vi "run.vi"(8 "error in (no error)":errorcluster, 11 "ScanModeDL091001Scaffold in":refnum<class "ImagingModeDL091001Scaffold.lvclass">) -> (0 "error out":errorcluster, 3 "ScanModeDL091001Scaffold out":refnum<class "ImagingModeDL091001Scaffold.lvclass">)   [LabVIEW 2010, in "ImagingModeDL091001Scaffold.lvclass"]
uses:
  ImagingModeDL091001Scaffold.lvclass
  internal_triggers_enum.ctl
  GenericImagingMode/GenericImagingMode/trigger_enum.ctl
  GenericImagingMode/GenericImagingMode/GenericImagingMode.lvclass
  Trajectory/GenericTrajectory/GenericTrajectory/GenericTrajectory.lvclass
  common/classes/ErrorController/ErrorController/class_data.vi
  common/classes/ErrorController/ErrorController/ErrorController.lvclass
panel:
  out "last trigger":T1
  out "statechart\nerror 2":errorcluster
  out "stage machine counter":i32
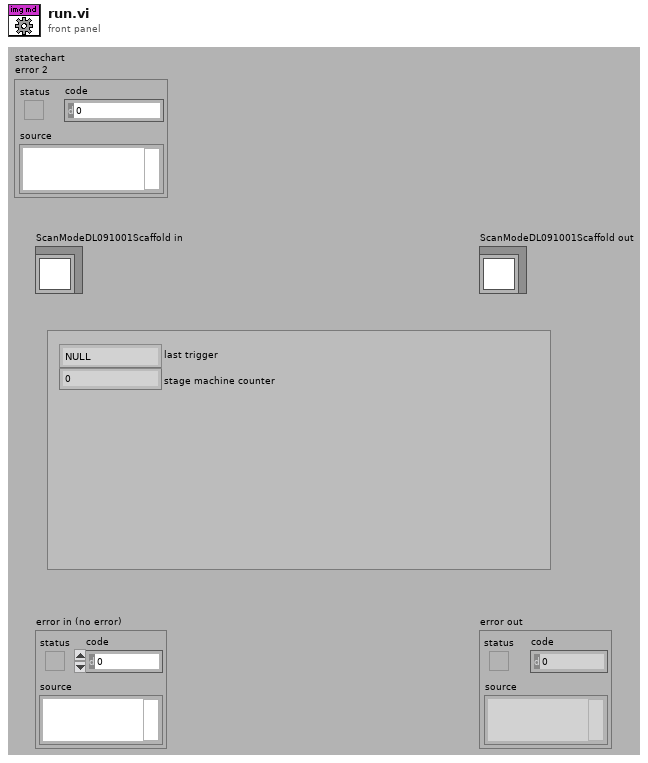
[diagram p1: front panel]
types:
  T1 = typedef "ImagingModeDL091001Scaffold.lvclass/internal_triggers_enum.ctl" = enum16{"NULL", "initialise", "terminate", "start sweep", "stop sweep", "update", "proceed", "draw overlay", "attach observer", "detach observer", "finish sweep"}
  T2 = typedef "GenericImagingMode.lvclass/trigger_enum.ctl" = enum16{"NULL", "proceed"}
  T3 = typedef "top-level_component_type_enum.ctl" = enum16{"undefined", "ImagingMode", "ScanHead", "DAQ", "ImageAssembler", "Display", "DataCollection", "Analyser", "Stimulator", "ExperimentController", "Instrument", "Stage"}
  T4 = typedef "main_trigger_enum.ctl" = enum16{"NULL", "initialise", "terminate", "start", "stop", "change objective", "change experimentController", "change imagingMode", "save notebook", "started saving", "finished saving", "expCtr ready", "expCtr missing", "imgMd ready", "imgMd missing", "scanHd ready", "scanHd missing", "DAQ ready", "DAQ missing", "imgAsm ready", "imgAsm missing", "dataColl ready", "dataColl missing", "display ready", "display missing", "analysr ready", "analysr missing", "instrmnt ready", "instrmnt missing", "stimltr ready", "stimltr missing", "stage ready", "stage missing"}
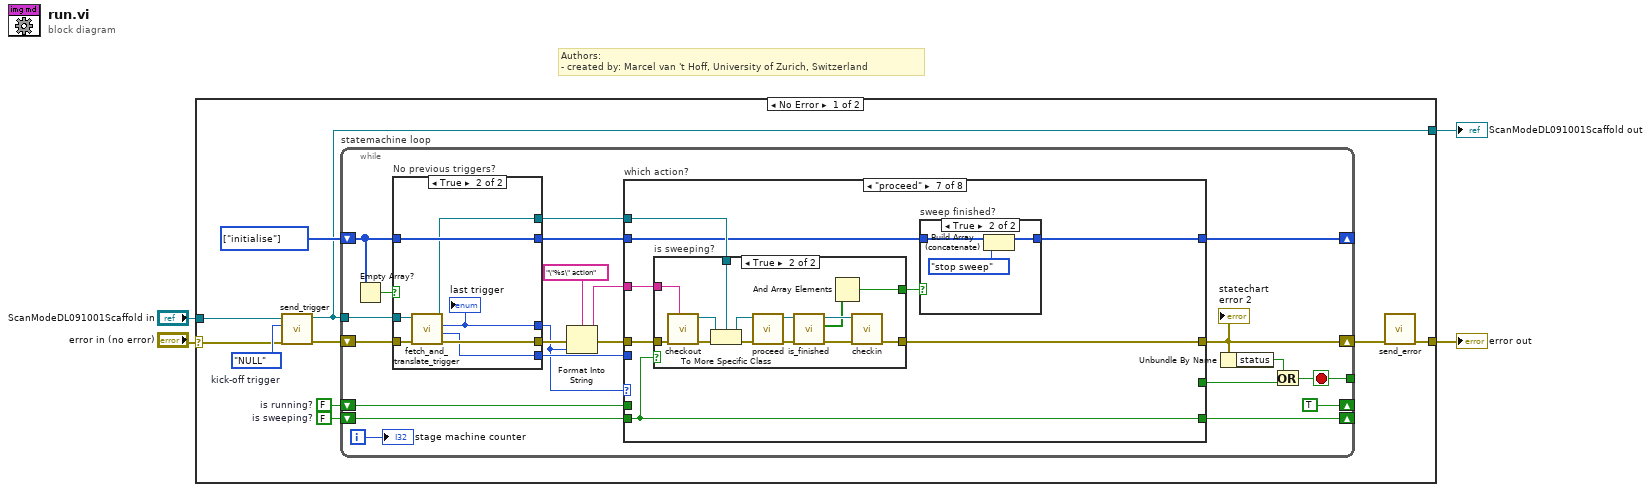
[diagram p0: block diagram]
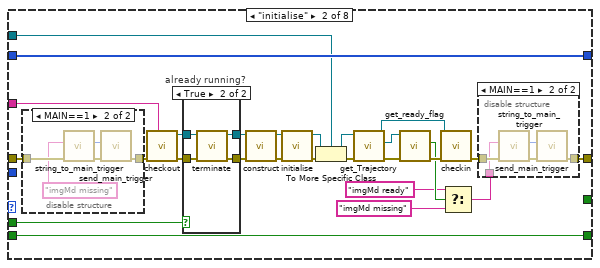
[diagram p3: hidden frame]
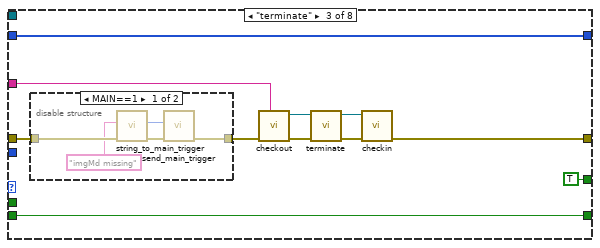
[diagram p7: hidden frame]
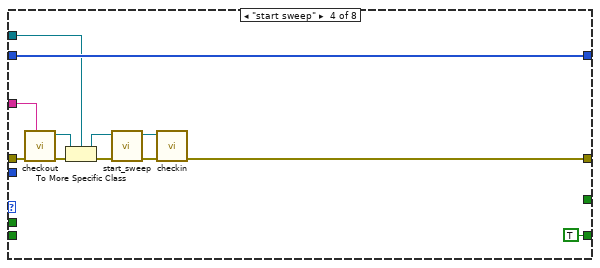
[diagram p9: hidden frame]
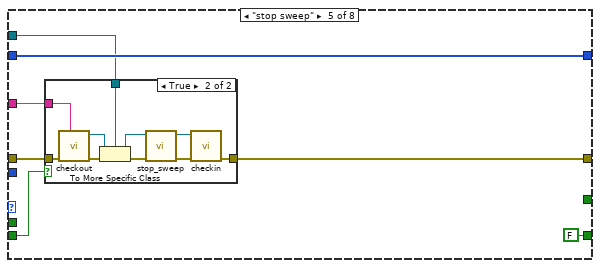
[diagram p10: hidden frame]
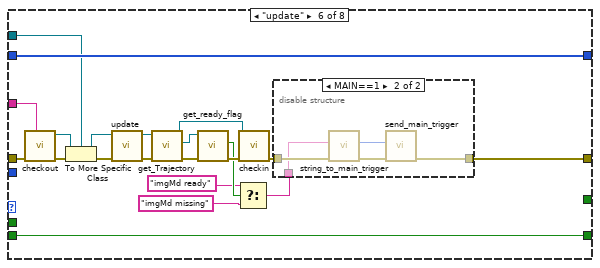
[diagram p12: hidden frame]
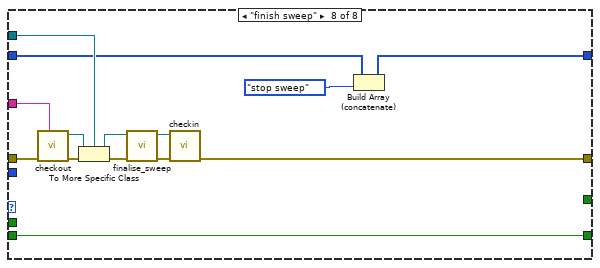
[diagram p16: hidden frame]
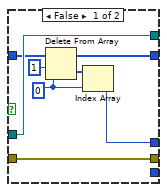
[diagram p17: hidden frame]
diagram:
  # "Authors: \n- created by: Marcel van 't Hoff, University of Zurich, Switzerland"
  n1 = case shown="No Error" "error in (no error)" {
    selector: "error in (no error)" -> [w12 w216]
    tunnel: [w6 w216] -> w3
    tunnel: "ScanModeDL091001Scaffold in" -> [w13 w215]
    tunnel: [w5 w215] -> w1
    frame No Error {
      w8 = FALSE  # is sweeping?
      w9 = FALSE  # is running?
      w10 = T1[] [enum."initialise"] items=["NULL", "initialise", "terminate", "start sweep", "stop sweep", "update", "proceed", "draw overlay", "attach observer", "detach observer", "finish sweep"]
      w14 = trigger_enum."NULL"  # kick-off trigger
      n2 = call-dynamic "send_trigger.vi"("error in (no error)"=w12, "message"=w14, "GenericScanMode in"=w13) -> ("error out"=w11:errorcluster, "GenericScanMode out"=w5:refnum<class "ImagingModeDL091001Scaffold.lvclass">)  [unwired: 7 in]
      n3 = while "statemachine loop" {
        shift-right: [w22] -> w7
        shift-left: w11 -> [w36]
        shift-right: [w27] -> _
        shift-left: w10 -> [w34]
        shift-right: [TRUE ("is running?")] -> _
        shift-left: w9 -> [w25]
        tunnel: [w19] -> _
        shift-right: [w16] -> _
        shift-left: w8 -> [w17]
        tunnel: w5 -> [w35]
        i -> [w18]
        stop <- w19 stop-if-true
        n4 = Empty Array?(array=w34) -> (empty?=w33:bool)
        n5 = case "No previous triggers?" shown="True" w33 {
          tunnel: w35 -> [w207 w211]
          tunnel: w36 -> [w205 w213]
          tunnel: [w207 w210] -> w26
          tunnel: [w203 w209] -> w15
          tunnel: [_ w208] -> w30
          tunnel: [w205 w212] -> w32
          tunnel: w34 -> [w206 w214]
          tunnel: [w202 w214] -> w28
          frame False {
            w200 = 0 ("index")
            n6 = Delete From Array(array=w206, length=1, index=w200) -> (deleted portion=w204:T1[], array with subset deleted=w202:T1[])
            n7 = Index Array(array=w204, index=w200) -> (element=w203:T1)
          }
          frame True {
            n8 = call-dynamic "fetch_and_translate_trigger.vi"("error in (no error)"=w213, "ImagingModeDL091001Scaffold in"=w211) -> ("error out"=w212:errorcluster, "sender TLC type"=w208:T3, "statechart trigger"=w209:T1, "ImagingModeDL091001Scaffold out"=w210:refnum<class "ImagingModeDL091001Scaffold.lvclass">)  [unwired: 6 in]
            "last trigger" <- w209
          }
        }
        n9 = Format Into String(format string="\"%s\" action", error in=w32, w15) -> (resulting string=w23:string, error out=w29:errorcluster)  [unwired: 1 in]
        n10 = case "which action?" shown="\"proceed\"" w15 {
          tunnel: w30 -> [_ _ _ _ _ _ _ _]
          tunnel: w29 -> [w38 w58 w87 w109 w119 w148 w165 w194]
          tunnel: w28 -> [w39 w66 w95 w113 w120 w152 w160 w188]
          tunnel: [w39 w66 w95 w113 w120 w152 w159 w187] -> w27
          tunnel: w26 -> [_ w51 _ w107 w117 w145 w162 w196]
          tunnel: [w38 w59 w92 w103 w116 w134 w164 w193] -> w22
          tunnel: w25 -> [_ w61 _ _ _ _ _ _]
          tunnel: w23 -> [_ w64 w91 w108 w118 w147 w163 w195]
          tunnel: [_ _ TRUE ("is running?") _ _ _ _ _] -> w20
          tunnel: w17 -> [w37 w56 w85 _ w114 w151 w166 w199]
          tunnel: [w37 w56 w85 TRUE ("is sweeping?") FALSE ("is sweeping?") w151 w166 w199] -> w16
          frame "NULL", Default {
          }
          frame "initialise" {
            n11 = disable-structure shown="MAIN==1" {
              disable-tunnel: [w67 w72] -> w57
              disable-tunnel: w58 -> [w67 w69]
              frame condition #0 (active) {
              }
              frame condition #1 {
                n12 = call "string_to_main_trigger.vi"("error in (no error)"=w69, "trigger string"="imgMd missing") -> ("error out"=w71:errorcluster, "main trigger"=w70:T4)  [unwired: 8 in]
                n13 = call "send_main_trigger.vi"("error in (no error)"=w71, "trigger"=w70) -> ("error out"=w72:errorcluster)  [unwired: 9 in]
              }
            }
            n14 = call "checkout.vi"("locked by?"=w64, "error in (no error)"=w57) -> ("error out"=w63:errorcluster, "GenericScanMode out"=w53:refnum<class "GenericImagingMode.lvclass">)  [unwired: 8 in]
            n15 = case "already running?" shown="True" w61 {
              tunnel: w63 -> [w79 w84]
              tunnel: w53 -> [w80 w82]
              tunnel: [w79 w83] -> w62
              tunnel: [w80 w81] -> w54
              frame False {
              }
              frame True {
                n16 = call-dynamic "terminate.vi"("error in (no error)"=w84, "GenericPlugin in"=w82) -> ("error out"=w83:errorcluster, "GenericPlugin out"=w81:refnum<class "GenericImagingMode.lvclass">)  [unwired: 8 out]
              }
            }
            n17 = call-dynamic "construct.vi"("error in (no error)"=w62, "GenericPlugin in"=w54) -> ("error out"=w65:errorcluster, "GenericPlugin out"=w55:refnum<class "GenericImagingMode.lvclass">)  [unwired: 8 in]
            n18 = call-dynamic "initialise.vi"("error in (no error)"=w65, "GenericPlugin in"=w55) -> ("error out"=w48:errorcluster, "GenericPlugin out"=w52:refnum<class "GenericImagingMode.lvclass">)  [unwired: 8 in]
            n19 = To More Specific Class(target class=w51, reference=w52, error in=w48) -> (specific class reference=w50:refnum<class "ImagingModeDL091001Scaffold.lvclass">, error out=w46:errorcluster)
            n20 = call-dynamic "get_Trajectory.vi"("error in (no error)"=w46, "ScanModeDL090923Scaffold in"=w50) -> ("error out"=w47:errorcluster, "Trajectory"=w49:refnum<class "GenericTrajectory.lvclass">, "ScanModeDL090923Scaffold out"=w43:refnum<class "ImagingModeDL091001Scaffold.lvclass">)  [unwired: 2 in, 5 out]
            n21 = call-dynamic "get_ready_flag.vi"("error in (no error)"=w47, "GenericTrajectory in"=w49) -> ("error out"=w45:errorcluster, "ready for initialisation?"=w42:bool)  [unwired: 7 in, 1 out]
            n22 = call-dynamic "checkin.vi"("error in (no error)"=w45, "GenericScanMode in"=w43) -> ("error out"=w60:errorcluster)  [unwired: 8 in, 1 out]
            n23 = Select(t="imgMd ready", s=w42, f="imgMd missing") -> (s? t:f=w44:string)
            n24 = disable-structure shown="MAIN==1" {
              disable-tunnel: [w73 w78] -> w59
              disable-tunnel: w60 -> [w73 w77]
              disable-tunnel: w44 -> [_ w74]
              frame condition #0 (active) {
              }
              frame condition #1 {
                n25 = call "string_to_main_trigger.vi"("error in (no error)"=w77, "trigger string"=w74) -> ("error out"=w76:errorcluster, "main trigger"=w75:T4)  [unwired: 8 in]
                n26 = call "send_main_trigger.vi"("error in (no error)"=w76, "trigger"=w75) -> ("error out"=w78:errorcluster)  [unwired: 9 in]
              }
            }
          }
          frame "terminate" {
            n27 = disable-structure shown="MAIN==1" {
              disable-tunnel: w87 -> [w99 w101]
              disable-tunnel: [w100 w101] -> w86
              frame condition #0 {
                n28 = call "string_to_main_trigger.vi"("error in (no error)"=w99, "trigger string"="imgMd missing") -> ("error out"=w98:errorcluster, "main trigger"=w97:T4)  [unwired: 8 in]
                n29 = call "send_main_trigger.vi"("error in (no error)"=w98, "trigger"=w97) -> ("error out"=w100:errorcluster)  [unwired: 9 in]
              }
              frame condition #1 (active) {
              }
            }
            n30 = call "checkout.vi"("locked by?"=w91, "error in (no error)"=w86) -> ("error out"=w93:errorcluster, "GenericScanMode out"=w90:refnum<class "GenericImagingMode.lvclass">)  [unwired: 8 in]
            n31 = call-dynamic "terminate.vi"("error in (no error)"=w93, "GenericPlugin in"=w90) -> ("error out"=w94:errorcluster, "GenericPlugin out"=w89:refnum<class "GenericImagingMode.lvclass">)  [unwired: 8 in]
            n32 = call-dynamic "checkin.vi"("error in (no error)"=w94, "GenericScanMode in"=w89) -> ("error out"=w92:errorcluster)  [unwired: 8 in, 1 out]
          }
          frame "start sweep" {
            n33 = call "checkout.vi"("locked by?"=w108, "error in (no error)"=w109) -> ("error out"=w111:errorcluster, "GenericScanMode out"=w106:refnum<class "GenericImagingMode.lvclass">)  [unwired: 8 in]
            n34 = To More Specific Class(target class=w107, reference=w106, error in=w111) -> (specific class reference=w105:refnum<class "ImagingModeDL091001Scaffold.lvclass">, error out=w112:errorcluster)
            n35 = call-dynamic "start_sweep.vi"("error in (no error)"=w112, "ScanModeDL091001Scaffold in"=w105) -> ("error out"=w110:errorcluster, "ScanModeDL091001Scaffold out"=w104:refnum<class "ImagingModeDL091001Scaffold.lvclass">)  [unwired: 8 in]
            n36 = call-dynamic "checkin.vi"("error in (no error)"=w110, "GenericScanMode in"=w104) -> ("error out"=w103:errorcluster)  [unwired: 8 in, 1 out]
          }
          frame "stop sweep" {
            n37 = case shown="True" w114 {
              tunnel: w119 -> [w121 w128]
              tunnel: w118 -> [_ w127]
              tunnel: w117 -> [_ w126]
              tunnel: [w121 w122] -> w116
              frame False {
              }
              frame True {
                n38 = call "checkout.vi"("locked by?"=w127, "error in (no error)"=w128) -> ("error out"=w130:errorcluster, "GenericScanMode out"=w125:refnum<class "GenericImagingMode.lvclass">)  [unwired: 8 in]
                n39 = To More Specific Class(target class=w126, reference=w125, error in=w130) -> (specific class reference=w124:refnum<class "ImagingModeDL091001Scaffold.lvclass">, error out=w131:errorcluster)
                n40 = call-dynamic "stop_sweep.vi"("error in (no error)"=w131, "ScanModeDL091001Scaffold in"=w124) -> ("error out"=w129:errorcluster, "ScanModeDL091001Scaffold out"=w123:refnum<class "ImagingModeDL091001Scaffold.lvclass">)  [unwired: 8 in]
                n41 = call-dynamic "checkin.vi"("error in (no error)"=w129, "GenericScanMode in"=w123) -> ("error out"=w122:errorcluster)  [unwired: 8 in, 1 out]
              }
            }
          }
          frame "update" {
            n42 = call "checkout.vi"("locked by?"=w147, "error in (no error)"=w148) -> ("error out"=w149:errorcluster, "GenericScanMode out"=w146:refnum<class "GenericImagingMode.lvclass">)  [unwired: 8 in]
            n43 = To More Specific Class(target class=w145, reference=w146, error in=w149) -> (specific class reference=w144:refnum<class "ImagingModeDL091001Scaffold.lvclass">, error out=w150:errorcluster)
            n44 = call-dynamic "update.vi"("error in (no error)"=w150, "ScanModeDL090923Scaffold in"=w144) -> ("error out"=w136:errorcluster, "ScanModeDL090923Scaffold out"=w137:refnum<class "ImagingModeDL091001Scaffold.lvclass">)  [unwired: 8 in]
            n45 = call-dynamic "get_Trajectory.vi"("error in (no error)"=w136, "ScanModeDL090923Scaffold in"=w137) -> ("error out"=w141:errorcluster, "Trajectory"=w142:refnum<class "GenericTrajectory.lvclass">, "ScanModeDL090923Scaffold out"=w135:refnum<class "ImagingModeDL091001Scaffold.lvclass">)  [unwired: 2 in, 5 out]
            n46 = call-dynamic "get_ready_flag.vi"("error in (no error)"=w141, "GenericTrajectory in"=w142) -> ("error out"=w140:errorcluster, "ready for initialisation?"=w139:bool)  [unwired: 7 in, 1 out]
            n47 = Select(t="imgMd ready", s=w139, f="imgMd missing") -> (s? t:f=w138:string)
            n48 = call-dynamic "checkin.vi"("error in (no error)"=w140, "GenericScanMode in"=w135) -> ("error out"=w143:errorcluster)  [unwired: 8 in, 1 out]
            n49 = disable-structure shown="MAIN==1" {
              disable-tunnel: [w153 w158] -> w134
              disable-tunnel: w143 -> [w153 w157]
              disable-tunnel: w138 -> [_ w155]
              frame condition #0 (active) {
              }
              frame condition #1 {
                n50 = call "string_to_main_trigger.vi"("error in (no error)"=w157, "trigger string"=w155) -> ("error out"=w156:errorcluster, "main trigger"=w154:T4)  [unwired: 8 in]
                n51 = call "send_main_trigger.vi"("error in (no error)"=w156, "trigger"=w154) -> ("error out"=w158:errorcluster)  [unwired: 9 in]
              }
            }
          }
          frame "proceed" {
            n52 = case "is sweeping?" shown="True" w166 {
              tunnel: w165 -> [w171 w183]
              tunnel: [w171 w182] -> w164
              tunnel: w163 -> [_ w181]
              tunnel: w162 -> [_ w178]
              tunnel: [_ w172] -> w161
              frame False {
              }
              frame True {
                n53 = call "checkout.vi"("locked by?"=w181, "error in (no error)"=w183) -> ("error out"=w184:errorcluster, "GenericScanMode out"=w180:refnum<class "GenericImagingMode.lvclass">)  [unwired: 8 in]
                n54 = To More Specific Class(target class=w178, reference=w180, error in=w184) -> (specific class reference=w179:refnum<class "ImagingModeDL091001Scaffold.lvclass">, error out=w185:errorcluster)
                n55 = call-dynamic "proceed.vi"("error in (no error)"=w185, "ScanModeDL091001Scaffold in"=w179) -> ("error out"=w177:errorcluster, "ScanModeDL091001Scaffold out"=w175:refnum<class "ImagingModeDL091001Scaffold.lvclass">)  [unwired: 8 in]
                n56 = call-dynamic "is_finished.vi"("error in (no error)"=w177, "ImagingModeDL090923Scaffold in"=w175) -> ("error out"=w176:errorcluster, "finished?"=w173:bool[], "ImagingModeDL090923Scaffold out"=w174:refnum<class "ImagingModeDL091001Scaffold.lvclass">)  [unwired: 7 in]
                n57 = And Array Elements(Boolean array=w173) -> (logical AND=w172:bool)
                n58 = call-dynamic "checkin.vi"("error in (no error)"=w176, "GenericScanMode in"=w174) -> ("error out"=w182:errorcluster)  [unwired: 8 in, 1 out]
              }
            }
            n59 = case "sweep finished?" shown="True" w161 {
              tunnel: w160 -> [w167 w170]
              tunnel: [w167 w169] -> w159
              frame False {
              }
              frame True {
                n60 = Build Array (concatenate)(w170, internal_triggers_enum."stop sweep" ("internal triggers enum")) -> (w169:T1[])
              }
            }
          }
          frame "finish sweep" {
            n61 = call "checkout.vi"("locked by?"=w195, "error in (no error)"=w194) -> ("error out"=w198:errorcluster, "GenericScanMode out"=w197:refnum<class "GenericImagingMode.lvclass">)  [unwired: 8 in]
            n62 = To More Specific Class(target class=w196, reference=w197, error in=w198) -> (specific class reference=w192:refnum<class "ImagingModeDL091001Scaffold.lvclass">, error out=w190:errorcluster)
            n63 = call-dynamic "finalise_sweep.vi"("error in (no error)"=w190, "ImagingModeDL091001Scaffold in"=w192) -> ("error out"=w189:errorcluster, "ImagingModeDL091001Scaffold out"=w191:refnum<class "ImagingModeDL091001Scaffold.lvclass">)  [unwired: 8 in]
            n64 = call-dynamic "checkin.vi"("error in (no error)"=w189, "GenericScanMode in"=w191) -> ("error out"=w193:errorcluster)  [unwired: 8 in, 1 out]
            n65 = Build Array (concatenate)(w188, internal_triggers_enum."stop sweep" ("internal triggers enum")) -> (w187:T1[])
          }
        }
        "statechart\nerror 2" <- w22
        n66 = Unbundle By Name(w22) -> ("status"=w21:bool)
        n67 = Or(x=w21, y=w20) -> (x .or. y?=w19:bool)
        "stage machine counter" <- w18
      }
      n68 = call "send_error.vi"("error in (no error)"=w7) -> ("error out"=w6:errorcluster)  [unwired: 10 in]
    }
    frame Error {
    }
  }
  "error out" <- w3
  "ScanModeDL091001Scaffold out" <- w1
